vi "Units Write.vi"(4 "error in (no error)":errorcluster, 5 "Value":string, 6 "Container State":T2, 7 "Display State In":T1) -> (0 "error out":errorcluster, 3 "Display State Out":T1)   [LabVIEW 2020, in "Filter (G3).xctl"]
uses:
  Filter (G3).xctl
  <vilib>/_xctls/Container State.ctl
  State.ctl
  <vilib>/_xctls/XControlSupport.lvlib
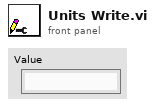
[diagram p1: front panel]
types:
  T1 = typedef "Filter (G3).xctl/State.ctl" = cluster{"Show cascade":bool, "Label color":u32, "TypeRef":refnum<vi>, "UnitsRef":refnum<vi>, "actions":string[]}
  T2 = typedef "XControlSupport.lvlib/Container State.ctl" = cluster{"Indicator?":bool, "Run Mode?":bool, " Refnum":refnum<vi>}
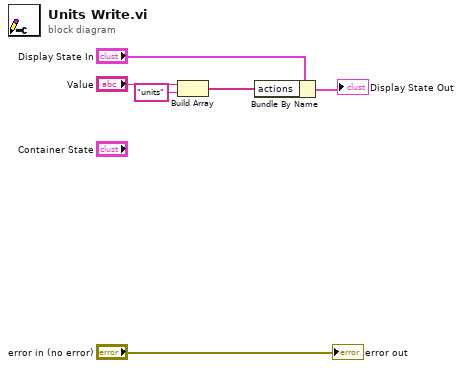
[diagram p0: block diagram]
diagram:
  n1 = Build Array("Value", "units" ("element")) -> (w2:string[])
  n2 = Bundle By Name(cluster="Display State In", "actions"=w2) -> (→"Display State Out":T1)
  "error out" <- "error in (no error)"
